vi "RoiConstructor.vi"() -> ()   [LabVIEW 2016]
doc: "Use this template to create a dialog box with event handling."
panel:
  in  "EraseROI":bool
  out "ROI Descriptor":T1 {"Contours"."Type" items=["No Selection", "Point", "Line", "Rectangle", "Oval", "Polygon", "Freehand Region", "Annulus", "Unused2", "Unused3", "Broken Line", "Freehand Line", "Rotated Rectangle"]}
  in  "ShowImg":bool
  in  "Exit":bool
  in  "DefROI":bool
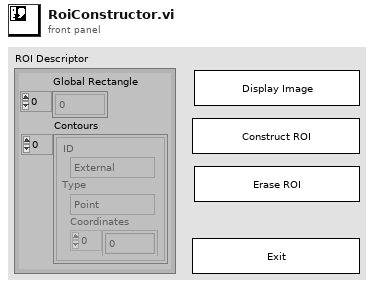
[diagram p1: front panel]
types:
  T1 = typedef "ROI Descriptor" = cluster{"Global Rectangle":i32[], "Contours":cluster{"ID":enum32{"External", "Internal"}, "Type":u32, "Coordinates":i32[]}[]}
  T2 = typedef "Image Type" = u32
  T3 = typedef "IMAQ Image.ctl" = refnum<image>
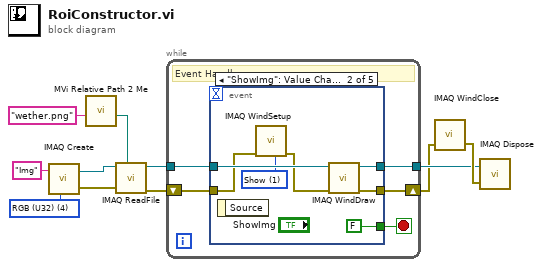
[diagram p0: block diagram]
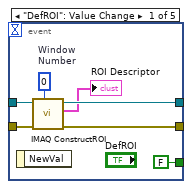
[diagram p2: hidden frame]
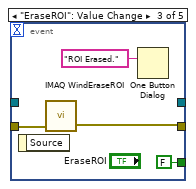
[diagram p3: hidden frame]
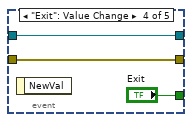
[diagram p4: hidden frame]
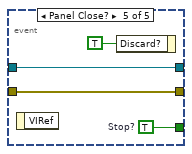
[diagram p5: hidden frame]
diagram:
  w9 = T2 4 items=["Grayscale (U8)", "Grayscale (I16)", "Grayscale (SGL)", "Complex (CSG)", "RGB (U32)", "HSL (U32)", "RGB (U64)", "Grayscale (U16)"] ("Image Type")
  n1 = call "IMAQ Create"("Image Name"="Img", "Image Type"=w9) -> ("New Image"=w10:T3, "error out"=w11:errorcluster)  [unwired: 3 in]
  n2 = call "MVi Relative Path 2 Me.vi"("Relative Path"="wether.png") -> ("Appended Dir"=w1:path)  [unwired: 5 in, 1 out]
  n3 = call "IMAQ ReadFile"("File Path"=w1, "error in (no error)"=w11, "Image"=w10) -> ("error out"=w4:errorcluster, "Image Out"=w5:T3)  [unwired: 4 in, 3 out]
  n4 = while {
    tunnel: w5 -> [w13]
    tunnel: [w12] -> w7
    shift-right: [w14] -> w3
    shift-left: w4 -> [w15]
    stop <- w16 stop-if-true
    # "Event Handler"
    n5 = event shown="[1] \"ShowImg\": Value Change" {
      selector: _ -> [_ _ _ _ _]
      dyn-events: _ -> [_ _ _ _ _]
      timeout: _ -> [_ _ _ _ _]
      tunnel: [FALSE ("Stop?") FALSE ("Stop?") FALSE ("Stop?") "Exit" w40] -> w16
      tunnel: [w19 w28 w32 w35 w39] -> w14
      tunnel: w15 -> [w22 w26 w33 w35 w39]
      tunnel: w13 -> [w21 w30 _ w36 w38]
      tunnel: [w18 w29 _ w36 w38] -> w12
      event "DefROI": Value Change {
        w20 = 0  # Window  Number
        n6 = event-data() -> ()  [unwired: 1 in, 1 out]
        n7 = call "IMAQ ConstructROI"("Window Number (-1...15)"=w20, "error in (no error)"=w22, "Image"=w21) -> ("error out"=w19:errorcluster, "ROI Descriptor Out"=→"ROI Descriptor":T1, "Image Out (duplicate)"=w18:T3)  [unwired: 5 in, 1 out]
      }
      event "ShowImg": Value Change {
        w24 = 1 items=["Hide", "Show", "No change"] ("Scrollbars (No change)")
        n8 = event-data() -> ()  [unwired: 1 in, 1 out]
        n9 = call "IMAQ WindSetup"("Scrollbars (No change)"=w24, "error in (no error)"=w26) -> ("error out"=w25:errorcluster)  [unwired: 9 in]
        n10 = call "IMAQ WindDraw"("error in (no error)"=w25, "Image"=w30) -> ("error out"=w28:errorcluster, "Image Out (duplicate)"=w29:T3)  [unwired: 8 in]
      }
      event "EraseROI": Value Change {
        n11 = event-data() -> ()  [unwired: 1 in, 1 out]
        n12 = call "IMAQ WindEraseROI"("error in (no error)"=w33) -> ("error out"=w32:errorcluster)  [unwired: 5 in]
        n13 = One Button Dialog(message="ROI Erased.") -> ()  [unwired: 1 in, 1 out]
      }
      event "Exit": Value Change {
        n14 = event-data() -> ()  [unwired: 1 in, 1 out]
      }
      event Panel Close? {
        w40 = TRUE  # Stop?
        n15 = event-data() -> ()  [unwired: 1 in, 1 out]
        n16 = event-data("Discard?"=TRUE) -> ()  [unwired: 1 in, 1 out]
      }
    }
  }
  n17 = call "IMAQ WindClose"("error in (no error)"=w3) -> ("error out"=w8:errorcluster)  [unwired: 5 in]
  n18 = call "IMAQ Dispose"("Image"=w7, "error in (no error)"=w8) -> ()  [unwired: 4 in, 1 out]
